vi "Lamp-IsConnected.vi"(8 "error in (no error)":errorcluster, 11 "Lamp in":refnum<vi>) -> (0 "error out":errorcluster, 2 "Connected":bool, 3 "Lamp out":refnum<vi>)   [LabVIEW 2016]
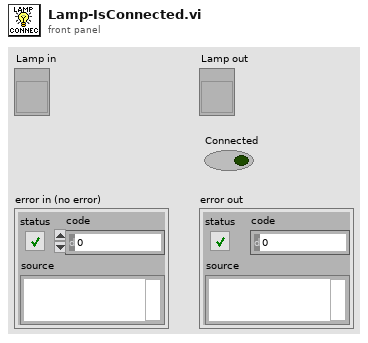
[diagram p1: front panel]
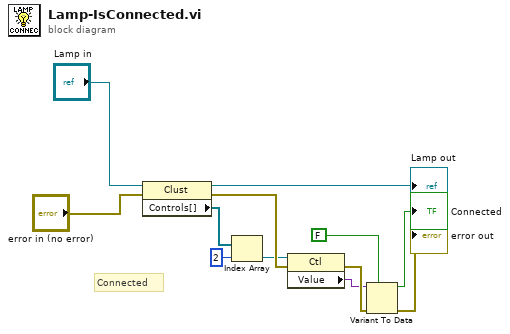
[diagram p0: block diagram]
diagram:
  # "Connected"
  n1 = property class="Clust"(reference="Lamp in", error in="error in (no error)") -> (reference out=→"Lamp out":refnum<vi>, error out=w9:errorcluster, "Controls[]"=w4:refnum<vi>[])
  n2 = Index Array(array=w4, index=2) -> (element=w6:refnum<vi>)
  n3 = property class="Ctl"(reference=w6, error in=w9) -> (error out=w8:errorcluster, "Value"=w7:variant)  [unwired: 1 out]
  n4 = Variant To Data(error in=w8, type=FALSE, Variant=w7) -> (data=→"Connected":bool, error out=→"error out":errorcluster)
